vi "S4GUI.vi"(7 "Tab ObsEng":enum32{"Obs", "CCD modes", "Eng"}(tab)) -> ()   [LabVIEW 2018] (continued)
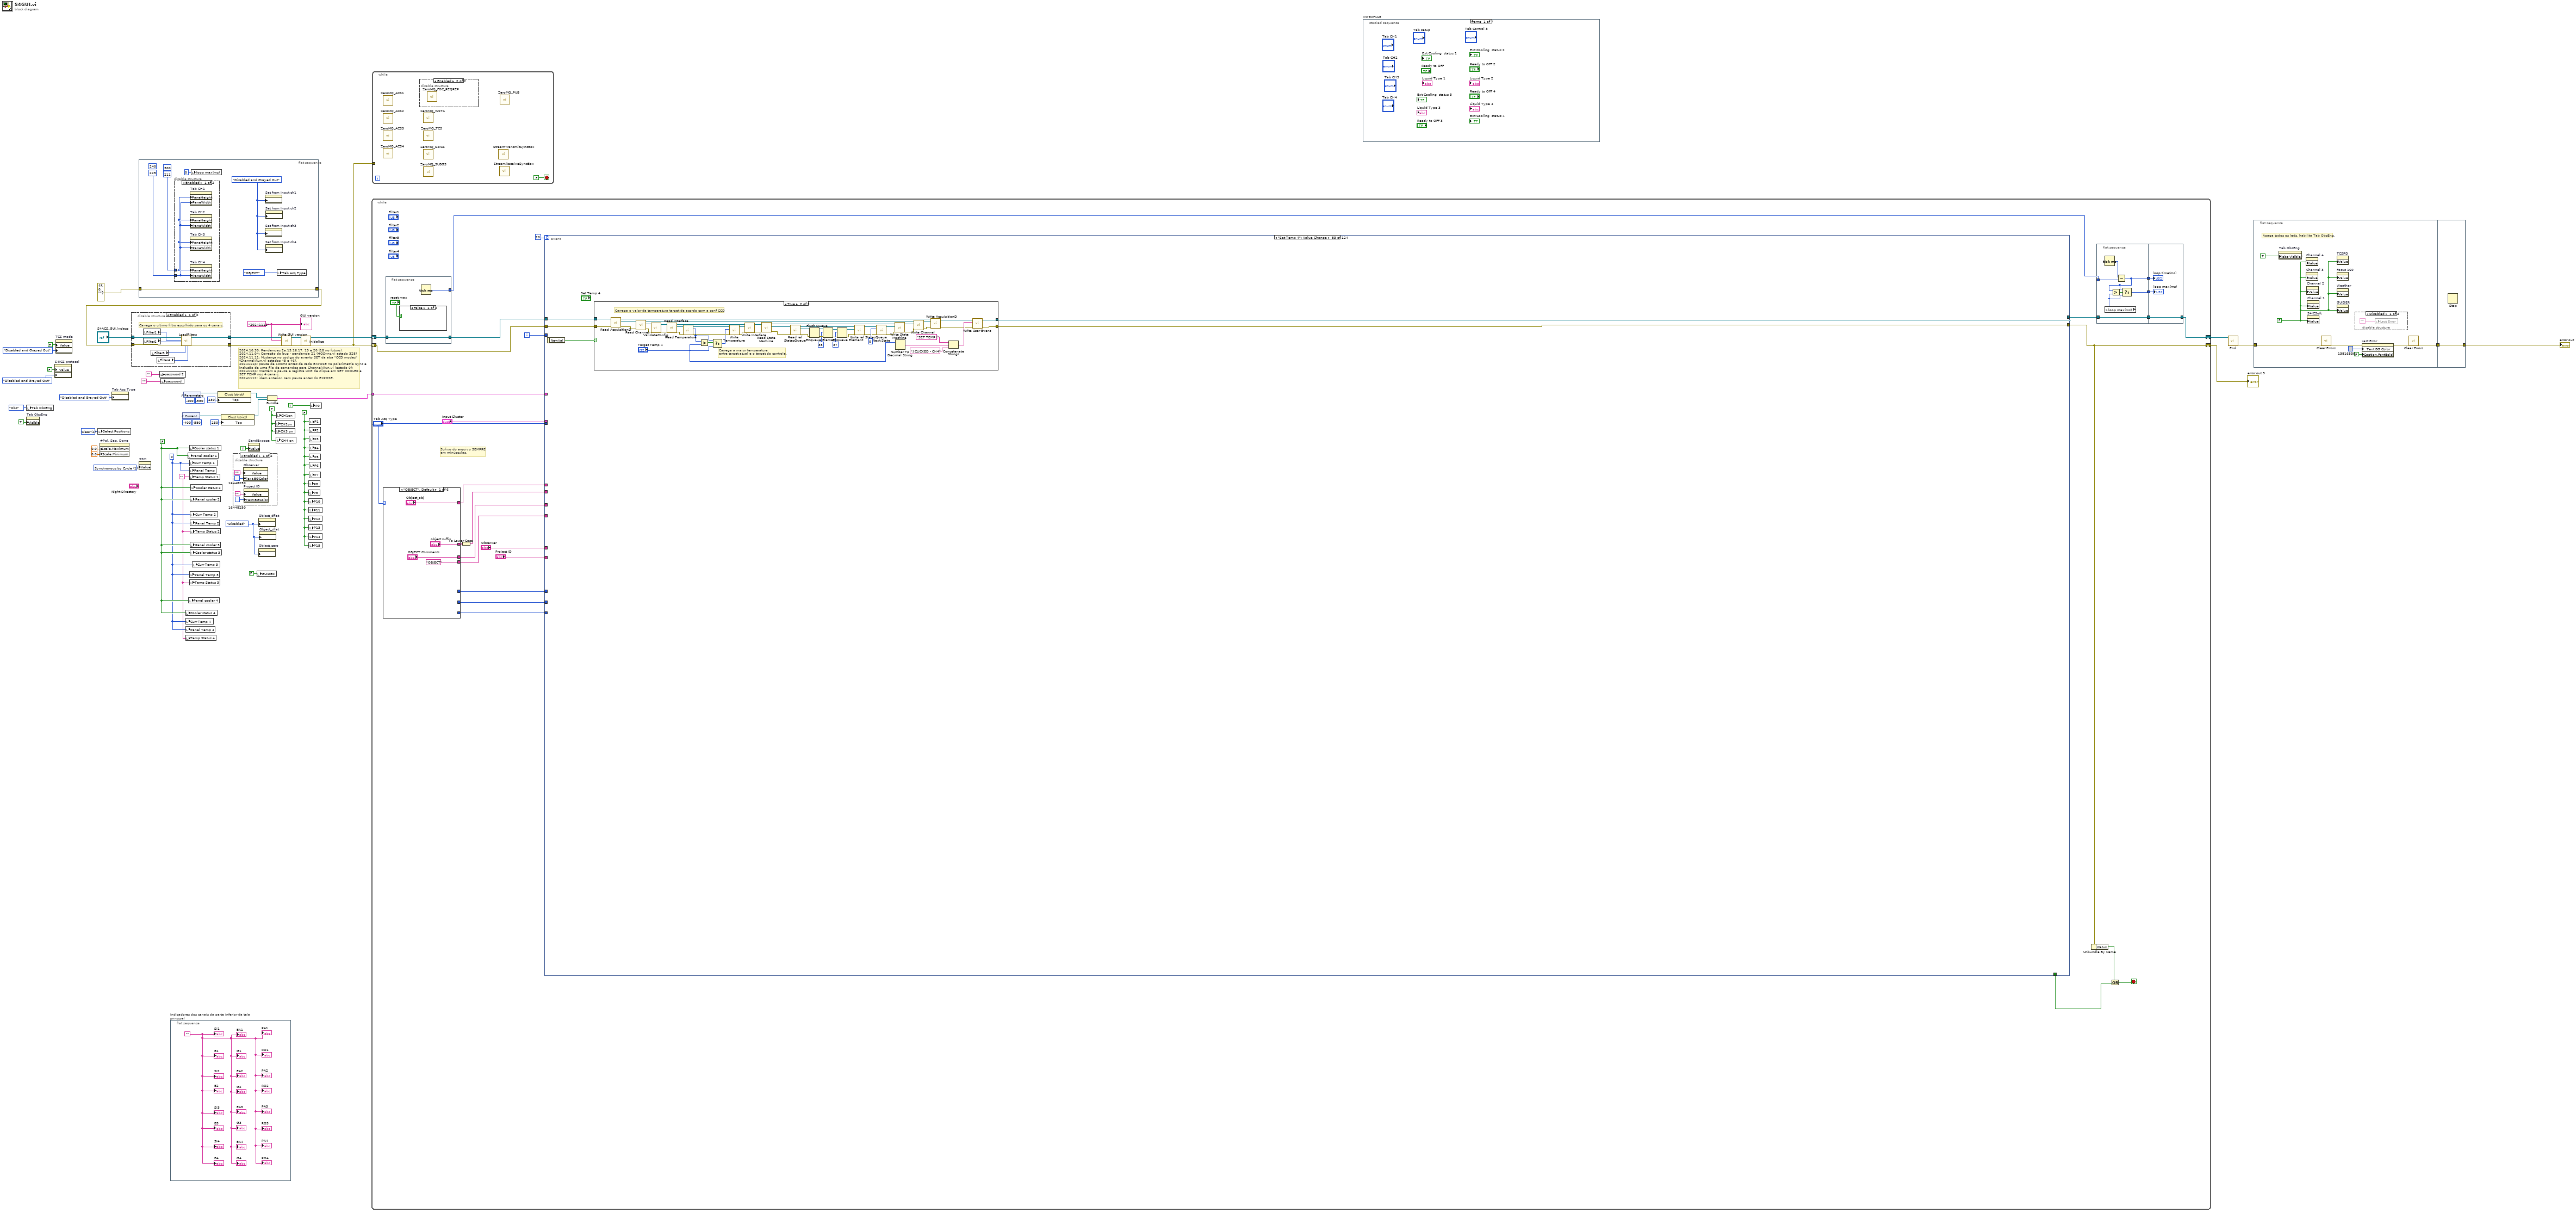
[diagram p0: block diagram]
diagram:
  w11 = "20241112" ("GUI version")
  w21 = TRUE ("CH1on")
  w26 = T12."Disabled" ("Disabled")
  (unwired) -580 ("Position:Top")
  (unwired) -400 ("Position:Top")
  w31 = "" ("Temp Status 1")
  w32 = i16 0 ("Curr Temp 1")
  w33 = FALSE ("Cooler status 1")
  w34 = u16 1 items=["Asynchronous", "Synchronous by Cycle"] ("SSM")
  (unwired) -400 ("Position:Top")
  (unwired) -580 ("Position:Top")
  w43 = u16 4 items=["All 16 positions", "First 8 positions", "First 4 positions", "1-4 & 9-12", "Clear", "Customized"] ("Select Positions")
  w25 = FALSE
  # "2024.10.30: Pendencias 2a,15,16,17, 19 e 20 (18 no futuro).\n2024.11.04: Correção do bug - pendencia 21 (HOSync.vi estado 328)\n2024.11.11: Mudança no código do evento SET da aba \"CCD modes\" \n(Channel:Run.vi estados 45 e 46).\n2024111p: pause de 100ms antes de cada EXPOSE na polarimetria Sync e \ninclusão de uma fila de comandos para Channel:Run.vi (estado 0);\n2024112p: mantém a pausa e registra LOG de clique em SET COOLER e \nSET TEMP nos 4 canais.\n20241112: idem anterior, sem pausa antes do EXPOSE."
  n1 = local write "Tab ObsEng"(enum32{"Obs", "CCD modes", "Eng"}."Obs" ("Tab ObsEng")) -> ()
  n2 = property on="Tab ObsEng" class="TabCtl (strict)"("Visible"=TRUE) -> ()  [unwired: 2 in, 2 out]
  n3 = property on="S4ICS protocol" class="Bool (strict)"("Value"=FALSE ("S4ICS protocol"), "DisabledEnum"=T12."Disabled and Grayed Out" ("Disabled")) -> ()  [unwired: 2 in, 2 out]
  n4 = property on="TCS mode" class="Bool (strict)"("Value"=TRUE ("TCS mode"), "DisabledEnum"=T12."Disabled and Grayed Out" ("Disabled")) -> ()  [unwired: 2 in, 2 out]
  n5 = local write "Select Positions"(w43) -> ()
  n6 = property on="#Pol. Seq. Done" class="Slide (strict)"("Scale.Maximum"=0.0 ("Scale.Range:Maximum"), "Scale.Minimum"=0.0 ("Scale.Range:Minimum")) -> ()  [unwired: 2 in, 2 out]
  n7 = property on="Tab Acq Type" class="TabCtl (strict)"("DisabledEnum"=T12."Disabled and Grayed Out" ("Disabled")) -> ()  [unwired: 2 in, 2 out]
  n8 = disable-structure shown="Enabled" {
    disable-tunnel: "S4ACS_GUI.lvclass" -> [w52 w54]
    disable-tunnel: w28 -> [w51 w53]
    disable-tunnel: [w46 w54] -> w15
    disable-tunnel: [w45 w53] -> w14
    frame Enabled {
      # "Carrega o ultimo filtro escolhido para os 4 canais."
      n9 = local read "Filter1"() -> (w50:u8)
      n10 = local read "Filter2"() -> (w49:u8)
      n11 = local read "Filter3"() -> (w48:u8)
      n12 = local read "Filter4"() -> (w47:u8)
      n13 = call-dynamic "LoadFilters.vi"("Filter 4"=w47, "Filter 3"=w48, "error in (no error)"=w51, "Filter 2"=w49, "Filter 1"=w50, "S4GUI in"=w52) -> ("error out"=w45:errorcluster, "S4GUI out"=w46:refnum<class "S4GUI.lvclass">)  [unwired: 4 in]
    }
    frame Disabled {
    }
  }
  n14 = flat-sequence {
    tunnel: errorcluster {"status"=FALSE, "code"=0, "source"=""} ("error in (no error)") -> [w57]
    tunnel: [w57] -> w28
    frame #0 {
      w56 = T12."Disabled and Grayed Out" ("Disabled")
      (unwired) u32 240 ("Tab Control Pane Dimension:Width")
      (unwired) u32 300 ("Tab Control Pane Dimension:Height")
      n15 = disable-structure shown="Enabled" {
        disable-tunnel: u32 211 ("Tab Control Pane Dimension:Height") -> [w62 _]
        disable-tunnel: u32 225 ("Tab Control Pane Dimension:Width") -> [w61 _]
        frame Enabled {
          n16 = property on="Tab CH1" class="TabCtl (strict)"("PaneHeight"=w62, "PaneWidth"=w61) -> ()  [unwired: 2 in, 2 out]
          n17 = property on="Tab CH2" class="TabCtl (strict)"("PaneHeight"=w62, "PaneWidth"=w61) -> ()  [unwired: 2 in, 2 out]
          n18 = property on="Tab CH3" class="TabCtl (strict)"("PaneHeight"=w62, "PaneWidth"=w61) -> ()  [unwired: 2 in, 2 out]
          n19 = property on="Tab CH4" class="TabCtl (strict)"("PaneHeight"=w62, "PaneWidth"=w61) -> ()  [unwired: 2 in, 2 out]
        }
        frame Disabled {
        }
      }
      n20 = local write "loop max(ms)"(u32 0 ("loop max(ms)")) -> ()
      n21 = property on="Set from Input ch1" class="Bool"("DisabledEnum"=w56) -> ()  [unwired: 2 in, 2 out]
      n22 = property on="Set from Input ch3" class="Bool"("DisabledEnum"=w56) -> ()  [unwired: 2 in, 2 out]
      n23 = property on="Set from Input ch2" class="Bool"("DisabledEnum"=w56) -> ()  [unwired: 2 in, 2 out]
      n24 = property on="Set from Input ch4" class="Bool"("DisabledEnum"=w56) -> ()  [unwired: 2 in, 2 out]
      n25 = local write "Tab Acq Type"(T1."OBJECT" ("Tab Acq Type")) -> ()
    }
  }
  n26 = property on="SSM" class="Ring (strict)"("Value"=w34) -> ()  [unwired: 2 in, 2 out]
  n27 = local write "password 2"("" ("password")) -> ()
  n28 = local write "password"("" ("password")) -> ()
  n29 = flat-sequence "Indicadores dos canais da parte inferior da tela principal" {
    frame #0 {
      w63 = ""
      "B1" <- w63
      "PA1" <- w63
      "RO1" <- w63
      "G1" <- w63
      "SI2" <- w63
      "PA2" <- w63
      "G2" <- w63
      "B2" <- w63
      "RO2" <- w63
      "EA2" <- w63
      "SI3" <- w63
      "EA3" <- w63
      "PA3" <- w63
      "B3" <- w63
      "G3" <- w63
      "RO3" <- w63
      "SI4" <- w63
      "EA4" <- w63
      "PA4" <- w63
      "B4" <- w63
      "G4" <- w63
      "RO4" <- w63
      "SI1" <- w63
      "EA1" <- w63
    }
  }
  n30 = control-ref of="Current Configuration"() -> (w41:refnum<vi>)
  n31 = control-ref of="Parameters"() -> (w38:refnum<vi>)
  n32 = local write "Cooler status 4"(w33) -> ()
  n33 = local write "Curr Temp 4"(w32) -> ()
  n34 = local write "Panel Temp 4"(w32) -> ()
  n35 = local write "Temp Status 4"(w31) -> ()
  n36 = local write "Panel cooler 1"(w33) -> ()
  n37 = local write "Panel cooler 4"(w33) -> ()
  n38 = local write "Cooler status 1"(w33) -> ()
  n39 = local write "Curr Temp 1"(w32) -> ()
  n40 = local write "Panel Temp"(w32) -> ()
  n41 = local write "Temp Status 1"(w31) -> ()
  n42 = local write "Panel Temp 3"(w32) -> ()
  n43 = local write "Temp Status 3"(w31) -> ()
  n44 = local write "Panel cooler 2"(w33) -> ()
  n45 = local write "Curr Temp 2"(w32) -> ()
  n46 = local write "Panel Temp 2"(w32) -> ()
  n47 = local write "Temp Status 2"(w31) -> ()
  n48 = local write "Panel cooler 3"(w33) -> ()
  n49 = local write "Cooler status 3"(w33) -> ()
  n50 = local write "Cooler status 2"(w33) -> ()
  n51 = local write "Curr Temp 3"(w32) -> ()
  n52 = property on="Property Node" class="Clust (strict)"(reference=w38, "Top"=230 ("Position:Top")) -> (reference out=w42:refnum<vi>)  [unwired: 1 in, 1 out]
  n53 = property on="Property Node" class="Clust (strict)"(reference=w41, "Top"=230 ("Position:Top")) -> (reference out=w40:refnum<vi>)  [unwired: 1 in, 1 out]
  n54 = disable-structure shown="Enabled" {
    frame Enabled {
      n55 = property on="Observer" class="Str"("Value"="" ("Observer"), "Text.BGColor"=u32 16448250) -> ()  [unwired: 2 in, 2 out]
      n56 = property on="Project ID" class="Str"("Value"="" ("Observer"), "Text.BGColor"=u32 16448250) -> ()  [unwired: 2 in, 2 out]
    }
    frame Disabled {
    }
  }
  n57 = property on="SendExpose" class="Bool (strict)"("Value"=TRUE ("ExtSync")) -> ()  [unwired: 2 in, 2 out]
  n58 = local write "GUIDER"(FALSE ("GUIDER")) -> ()
  n59 = property on="Object_dflat" class="Str"("DisabledEnum"=w26) -> ()  [unwired: 2 in, 2 out]
  n60 = property on="Object_zero" class="Str"("DisabledEnum"=w26) -> ()  [unwired: 2 in, 2 out]
  n61 = property on="Object_sflat" class="Str"("DisabledEnum"=w26) -> ()  [unwired: 2 in, 2 out]
  n62 = Bundle("Parameters"=w42, "Current Configuration"=w40) -> (w39:T13)  [unwired: 1 in]
  n63 = local write "CH2on"(w21) -> ()
  n64 = local write "CH3 on"(w21) -> ()
  n65 = local write "CH4 on"(w21) -> ()
  n66 = local write "CH1on"(w21) -> ()
  n67 = call-dynamic "Write GUI version.vi"("error in (no error)"=w14, "GUI version"=w11, "S4GUI in"=w15) -> ("error out"=w12:errorcluster, "S4GUI out"=w13:refnum<class "S4GUI.lvclass">)  [unwired: 7 in]
  n68 = call-dynamic "Initialize.vi"("error in (no error)"=w12, "S4ACS_GUI in"=w13) -> ("error out"=w5:errorcluster, "S4ACS_GUI out"=w6:refnum<class "S4GUI.lvclass">)  [unwired: 8 in]
  n69 = local write "P8"(w25) -> ()
  n70 = local write "P9"(w25) -> ()
  n71 = local write "P10"(w25) -> ()
  n72 = local write "P11"(w25) -> ()
  n73 = local write "P12"(w25) -> ()
  n74 = local write "P13"(w25) -> ()
  n75 = local write "P14"(w25) -> ()
  n76 = local write "P15"(w25) -> ()
  n77 = local write "P1"(w25) -> ()
  n78 = local write "P2"(w25) -> ()
  n79 = local write "P3"(w25) -> ()
  n80 = local write "P4"(w25) -> ()
  n81 = local write "P5"(w25) -> ()
  n82 = local write "P6"(w25) -> ()
  n83 = local write "P7"(w25) -> ()
  n84 = local write "P0"(TRUE ("P0")) -> ()
  n85 = while {
    shift-right: [w84] -> w44
    shift-left: w6 -> [w87]
    shift-right: [w71] -> w20
    shift-left: w5 -> [w95]
    tunnel: w39 -> [w92]
    i -> [w77]
    stop <- w68 stop-if-true
    # "Sufixo do arquivo SEMPRE\nem minúsculas."
    n86 = case shown="\"OBJECT\", Default" "Tab Acq Type" {
      tunnel: ["object suffix" "dflat suffix" "sflat suffix" "dark suffix" "zero suffix" "focus suffix"] -> w79
      tunnel: ["OBJECT Comments" "DFLAT Comments" "SFLAT Comments" "DARK Comments" "ZERO Comments" "FOCUS Comments"] -> w93
      tunnel: ["OBJECT" "FLAT" "FLAT" "DARK" "ZERO" "FOCUS"] -> w90
      tunnel: ["Object_obj" "DOMEFLAT" "SKYFLAT" "Object_dark" "ZERO" "Object_focus"] -> w89
      tunnel: [_ _ _ _ _ "Start focus"] -> w76
      tunnel: [_ _ _ _ _ "Step focus"] -> w74
      tunnel: [_ _ _ _ _ "#steps"] -> w75
      frame "OBJECT", Default {
      }
      frame "DFLAT" {
      }
      frame "SFLAT" {
      }
      frame "DARK" {
      }
      frame "ZERO" {
      }
      frame "FOCUS" {
      }
    }
    n87 = flat-sequence {
      tunnel: w87 -> [w108]
      tunnel: [w108] -> w86
      tunnel: [w107] -> w83
      frame #0 {
        n88 = case shown="False" "reset max" {
          frame False {
          }
          frame True {
            n89 = local write "loop max(ms)"(u32 0 ("loop max(ms)")) -> ()
          }
        }
        n90 = Tick Count (ms)() -> (millisecond timer value=w107:u32)
      }
    }
    n91 = To Lower Case(string=w79) -> (all lower case string=w78:string)
    n92 = event shown="[82] \"Set Temp 4\": Value Change" {
      selector: _ -> [_ _ _ _ _ _ _ _ _ _ _ _ _ _ _ _ _ _ _ _ _ _ _ _ _ _ _ _ _ _ _ _ _ _ _ _ _ _ _ _ _ _ _ _ _ _ _ _ _ _ _ _ _ _ _ _ _ _ _ _ _ _ _ _ _ _ _ _ _ _ _ _ _ _ _ _ _ _ _ _ _ _ _ _ _ _ _ _ _ _ _ _ _ _ _ _ _ _ _ _ _ _ _ _ _ _ _ _ _ _ _ _ _ _ _ _ _ _ _ _ _ _ _ _]
      dyn-events: _ -> [_ _ _ _ _ _ _ _ _ _ _ _ _ _ _ _ _ _ _ _ _ _ _ _ _ _ _ _ _ _ _ _ _ _ _ _ _ _ _ _ _ _ _ _ _ _ _ _ _ _ _ _ _ _ _ _ _ _ _ _ _ _ _ _ _ _ _ _ _ _ _ _ _ _ _ _ _ _ _ _ _ _ _ _ _ _ _ _ _ _ _ _ _ _ _ _ _ _ _ _ _ _ _ _ _ _ _ _ _ _ _ _ _ _ _ _ _ _ _ _ _ _ _ _]
      timeout: 20 -> [_ _ _ _ _ _ _ _ _ _ _ _ _ _ _ _ _ _ _ _ _ _ _ _ _ _ _ _ _ _ _ _ _ _ _ _ _ _ _ _ _ _ _ _ _ _ _ _ _ _ _ _ _ _ _ _ _ _ _ _ _ _ _ _ _ _ _ _ _ _ _ _ _ _ _ _ _ _ _ _ _ _ _ _ _ _ _ _ _ _ _ _ _ _ _ _ _ _ _ _ _ _ _ _ _ _ _ _ _ _ _ _ _ _ _ _ _ _ _ _ _ _ _ _]
      tunnel: w86 -> [w179 w2139 w2298 w2328 w2334 w2356 w2378 w2549 w2557 w2636 w2657 w2729 w2800 w2901 w2916 w3042 w3221 w3253 w3285 w3317 w3352 w3387 w3422 w3457 w3460 w3494 w3636 w3697 w4204 w4283 w4355 w4426 w4499 w4550 w4591 w5020 w5026 w5141 w6423 w6694 w6899 w7100 w7313 w7532 w7547 w7755 w7917 w8084 w8251 w8410 w8430 w8450 w8470 w8491 w8556 w8621 w8686 w8751 w8788 w8816 w8844 w8873 w8946 w9076 w9110 w9169 w9228 w9287 w9346 w9366 w9393 w9409 w9430 w9460 w9490 w9520 w9555 w9594 w9634 w9673 w9734 w9795 w9856 w9922 w9942 w9957 w9972 w9987 w10002 w10017 w10032 w10047 w10078 w10107 w10131 w10173 w10207 w10234 w10257 w10285 w10305 w10320 w10340 w10423 w10751 w10782 w10842 w10862 w10877 w10897 w10917 w10937 w10952 w10972 w10992 w11012 w11027 w11047 w11067 w11087 w11102 w11122 w11142 w11162]
      tunnel: w95 -> [w178 w2140 w2296 w2327 w2333 w2355 w2377 w2548 w2556 w2635 w2656 w2728 w2801 w2900 w2907 w3033 w3220 w3252 w3284 w3316 w3351 w3386 w3421 w3456 w3468 w3495 w3635 w3696 w4203 w4282 w4354 w4422 w4498 w4548 w4590 w5019 w5025 w5140 w6422 w6693 w6898 w7099 w7306 w7530 w7546 w7753 w7916 w8082 w8250 w8411 w8431 w8451 w8471 w8490 w8555 w8620 w8685 w8749 w8786 w8814 w8842 w8872 w8945 w9075 w9109 w9168 w9227 w9286 w9345 w9365 w9392 w9408 w9429 w9459 w9489 w9518 w9554 w9593 w9633 w9672 w9733 w9794 w9855 w9921 w9941 w9956 w9971 w9986 w10001 w10016 w10031 w10046 w10077 w10106 w10130 w10172 w10206 w10233 w10256 w10284 w10304 w10319 w10339 w10424 w10750 w10781 w10841 w10861 w10876 w10896 w10916 w10936 w10951 w10971 w10991 w11011 w11026 w11046 w11066 w11086 w11101 w11121 w11141 w11161]
      tunnel: [w139 w2102 w2290 w2315 w2335 w2357 w2379 w2536 w2574 w2635 w2674 w2746 w2818 w2887 w2914 w3040 w3131 w3239 w3271 w3303 w3342 w3377 w3412 w3447 w3468 w3480 w3600 w3684 w4123 w4280 w4352 w4417 w4496 w4551 w4585 w5018 w5022 w5106 w6484 w6687 w6892 w7093 w7307 w7531 w7539 w7749 w7926 w8093 w8260 w8409 w8429 w8449 w8469 w8489 w8554 w8619 w8684 w8750 w8787 w8815 w8843 w8877 w8950 w9077 w9108 w9167 w9226 w9285 w9344 w9364 w9391 w9407 w9428 w9458 w9488 w9547 w9585 w9624 w9663 w9671 w9732 w9793 w9854 w9920 w9940 w9955 w9970 w9985 w10000 w10015 w10030 w10045 w10062 w10104 w10129 w10171 w10205 w10232 w10255 w10267 w10287 w10307 w10323 w10347 w10758 w10783 w10824 w10844 w10864 w10882 w10899 w10919 w10939 w10955 w10974 w10994 w11014 w11030 w11049 w11069 w11089 w11105 w11124 w11144] -> w71
      tunnel: [w138 _ _ _ _ _ _ _ _ _ _ _ _ _ _ _ _ _ _ _ _ _ _ _ _ _ _ _ _ _ _ _ _ _ _ _ _ _ _ _ _ _ _ _ _ _ _ _ _ _ _ _ _ _ _ _ _ _ _ _ _ _ _ _ _ _ _ _ _ _ _ _ _ _ _ _ _ _ _ _ _ _ _ _ _ _ _ _ _ _ _ _ _ _ _ _ _ _ _ _ _ _ _ _ _ _ _ _ _ _ _ _ _ _ _ _ _ _ _ _ _ _ _ _] -> w69
      tunnel: w78 -> [_ _ _ _ _ _ _ _ _ _ _ _ _ _ _ _ _ _ _ _ _ _ _ _ _ _ _ _ _ _ _ _ _ _ w4584 _ _ _ _ w6692 w6896 _ w7311 _ w7544 w7762 w7925 w8092 w8259 _ _ _ _ _ _ _ _ _ _ _ _ _ _ _ _ _ _ _ _ _ _ _ _ _ _ _ _ _ _ _ _ _ _ _ _ _ _ _ _ _ _ _ _ _ _ _ _ _ _ _ _ _ _ _ _ _ _ _ _ _ _ _ _ _ _ _ _ _ _ _ _ _ _ _]
      tunnel: w93 -> [_ _ _ _ _ _ _ _ _ _ _ _ _ _ _ _ _ _ _ _ _ _ _ _ _ _ _ _ _ _ _ _ _ _ w4583 _ _ _ _ w6691 _ w7097 w7310 _ w7543 w7761 w7924 w8091 w8258 _ _ _ _ _ _ _ _ _ _ _ _ _ _ _ _ _ _ _ _ _ _ _ _ _ _ _ _ _ _ _ _ _ _ _ _ _ _ _ _ _ _ _ _ _ _ _ _ _ _ _ _ _ _ _ _ _ _ _ _ _ _ _ _ _ _ _ _ _ _ _ _ _ _ _]
      tunnel: w92 -> [_ _ _ _ _ _ _ _ _ _ _ _ _ _ _ _ _ _ _ _ _ _ _ _ w3461 _ _ _ _ _ _ _ _ _ _ _ _ _ _ _ _ _ _ _ _ _ _ _ _ _ _ _ _ _ _ _ _ _ _ _ _ _ _ _ _ _ _ _ _ _ _ _ _ _ _ _ _ _ _ _ _ _ _ _ _ _ _ _ _ _ _ _ _ _ _ _ _ _ _ _ _ _ _ _ _ _ _ _ _ _ _ _ _ _ _ _ _ _ _ _ _ _ _ _]
      tunnel: [w140 w2104 w2289 w2316 w2336 w2358 w2380 w2537 w2575 w2636 w2675 w2747 w2819 w2878 w2915 w3041 w3133 w3230 w3262 w3294 w3319 w3354 w3389 w3424 w3460 w3479 w3601 w3685 w4124 w4281 w4353 w4418 w4497 w4552 w4565 w5017 w5021 w5107 w6483 w6688 w6893 w7094 w7308 w7532 w7540 w7750 w7923 w8090 w8257 w8408 w8428 w8448 w8468 w8488 w8553 w8618 w8683 w8748 w8785 w8813 w8841 w8875 w8948 w9078 w9107 w9166 w9225 w9284 w9343 w9363 w9383 w9406 w9427 w9457 w9487 w9546 w9586 w9625 w9664 w9670 w9731 w9792 w9853 w9913 w9936 w9951 w9966 w9981 w9996 w10011 w10026 w10041 w10061 w10079 w10116 w10140 w10188 w10218 w10243 w10266 w10286 w10306 w10321 w10348 w10759 w10784 w10823 w10843 w10863 w10880 w10898 w10918 w10938 w10953 w10973 w10993 w11013 w11028 w11048 w11068 w11088 w11103 w11123 w11143] -> w85
      tunnel: "Input Cluster" -> [_ _ _ _ _ _ _ _ _ _ _ _ _ _ _ _ _ _ _ _ _ _ _ _ w3459 _ _ _ _ _ _ _ _ _ _ _ _ _ _ _ _ _ _ _ _ _ _ _ _ _ _ _ _ _ _ _ _ _ _ _ _ _ _ _ _ _ _ _ _ _ _ _ _ _ _ _ _ _ _ _ _ _ _ _ _ _ _ _ _ _ _ _ _ _ _ _ _ _ _ _ _ _ _ _ _ _ _ _ _ _ _ _ _ _ _ _ _ _ _ _ _ _ _ _]
      tunnel: w90 -> [_ _ _ _ _ _ _ _ _ _ _ _ _ _ _ _ _ _ _ _ _ _ _ _ _ _ _ _ _ _ _ _ _ _ w4582 _ _ _ _ w6689 w6894 w7095 w7309 _ w7541 w7760 w7922 w8088 w8256 _ _ _ _ _ _ _ _ _ _ _ _ _ _ _ _ _ _ _ _ _ _ _ _ _ _ _ _ _ _ _ _ _ _ _ _ _ _ _ _ _ _ _ _ _ _ _ _ _ _ _ _ _ _ _ _ _ _ _ _ _ _ _ _ _ _ _ _ _ _ _ _ _ _ _]
      tunnel: w89 -> [_ _ _ _ _ _ _ _ _ _ _ _ _ _ _ _ _ _ _ _ _ _ _ _ _ _ _ _ _ _ _ _ _ _ w4581 _ _ _ _ _ w6897 w7098 w7312 _ w7545 w7759 w7921 w8089 w8255 _ _ _ _ _ _ _ _ _ _ _ _ _ _ _ _ _ _ _ _ _ _ _ _ _ _ _ _ _ _ _ _ _ _ _ _ _ _ _ _ _ _ _ _ _ _ _ _ _ _ _ _ _ _ _ _ _ _ _ _ _ _ _ _ _ _ _ _ _ _ _ _ _ _ _]
      tunnel: "Observer" -> [_ _ _ _ _ _ _ _ _ _ _ _ _ _ _ _ _ _ _ _ _ _ _ _ _ _ _ _ _ _ _ _ _ _ w4580 _ _ w5112 w6432 w6690 w6895 w7096 _ _ w7542 w7758 w7920 w8087 w8254 _ _ _ _ _ _ _ _ _ _ _ _ _ _ _ _ _ _ _ _ _ _ _ _ _ _ _ _ _ _ _ _ _ _ _ _ _ _ _ _ _ _ _ _ _ _ _ _ _ _ _ _ _ _ _ _ _ _ _ _ _ _ _ _ _ _ _ _ _ _ _ _ _ _ _]
      tunnel: w77 -> [w159 _ _ _ _ _ _ _ _ _ _ _ _ _ _ _ _ _ _ _ _ _ _ _ _ _ _ _ _ _ _ _ _ _ _ _ _ _ _ _ _ _ _ _ _ _ _ _ _ _ _ _ _ _ _ _ _ _ _ _ _ _ _ _ _ _ _ _ _ _ _ _ _ _ _ _ _ _ _ _ _ _ _ _ _ _ _ _ _ _ _ _ _ _ _ _ _ _ _ _ _ _ _ _ _ _ _ _ _ _ _ _ _ _ _ _ _ _ _ _ _ _ _ _]
      tunnel: "Tab Acq Type" -> [_ _ _ _ _ _ _ _ _ _ _ _ _ _ _ _ _ _ _ _ _ _ _ _ _ _ _ _ _ _ _ _ _ _ w4572 _ _ _ _ _ _ w7084 _ _ _ w7747 w7911 w8078 w8244 _ _ _ _ _ _ _ _ _ _ _ _ _ _ _ _ _ _ _ _ _ _ _ _ _ _ _ _ _ _ _ _ _ _ _ _ _ _ _ _ _ _ _ _ _ _ _ _ _ _ _ _ _ _ _ _ _ _ _ _ _ _ _ _ _ _ _ _ _ _ _ _ _ _ _]
      tunnel: w76 -> [_ _ _ _ _ _ _ _ _ _ _ _ _ _ _ _ _ _ _ _ _ _ _ _ _ _ _ _ _ _ _ _ _ _ w4571 _ _ _ _ _ _ _ _ _ _ w7746 w7910 w8077 w8243 _ _ _ _ _ _ _ _ _ _ _ _ _ _ _ _ _ _ _ _ _ _ _ _ _ _ _ _ _ _ _ _ _ _ _ _ _ _ _ _ _ _ _ _ _ _ _ _ _ _ _ _ _ _ _ _ _ _ _ _ _ _ _ _ _ _ _ _ _ _ _ _ _ _ _]
      tunnel: w75 -> [_ _ _ _ _ _ _ _ _ _ _ _ _ _ _ _ _ _ _ _ _ _ _ _ _ _ _ _ _ _ _ _ _ _ w4569 _ _ _ _ _ _ _ _ _ _ w7744 w7908 w8075 w8241 _ _ _ _ _ _ _ _ _ _ _ _ _ _ _ _ _ _ _ _ _ _ _ _ _ _ _ _ _ _ _ _ _ _ _ _ _ _ _ _ _ _ _ _ _ _ _ _ _ _ _ _ _ _ _ _ _ _ _ _ _ _ _ _ _ _ _ _ _ _ _ _ _ _ _]
      tunnel: w74 -> [_ _ _ _ _ _ _ _ _ _ _ _ _ _ _ _ _ _ _ _ _ _ _ _ _ _ _ _ _ _ _ _ _ _ w4570 _ _ _ _ _ _ _ _ _ _ w7745 w7909 w8076 w8242 _ _ _ _ _ _ _ _ _ _ _ _ _ _ _ _ _ _ _ _ _ _ _ _ _ _ _ _ _ _ _ _ _ _ _ _ _ _ _ _ _ _ _ _ _ _ _ _ _ _ _ _ _ _ _ _ _ _ _ _ _ _ _ _ _ _ _ _ _ _ _ _ _ _ _]
      tunnel: "Project ID" -> [_ _ _ _ _ _ _ _ _ _ _ _ _ _ _ _ _ _ _ _ _ _ _ _ _ _ _ _ _ _ _ _ _ _ _ _ _ w5111 w6431 _ _ _ _ _ _ _ _ _ _ _ _ _ _ _ _ _ _ _ _ _ _ _ _ _ _ _ _ _ _ _ _ _ _ _ _ _ _ _ _ _ _ _ _ _ _ _ _ _ _ _ _ _ _ _ _ _ _ _ _ _ _ _ _ _ _ _ _ _ _ _ _ _ _ _ _ _ _ _ _ _ _ _ _ _]
      event Timeout {
        # "2024.07.02: Mostra as publicações das aplicações."
        # "Trata as tarefas para atender \naos clientes: Publisher"
        # "Conteudo dos indicadores"
        # "Status dos indicadores: Habilitado ou Desab."
        # "Obtém os valores de status dos\ndispositivos de cada servidor para\napresentar nos indicadores da GUI."
        # "Trata as tarefas individuais de \ncada servidor (ACS1,...,ACS4, \nICS, TCS, Focus,Weather)"
        # "Determina a sequência de\ntarefas dos servidores\npara uma observação, de \nacordo com o modo de \noperação (disparado com \nos botões START)"
        # "execução dos botões\n no modo sincrono."
        # "execução dos botões\n no modo assincrono."
        n93 = event-data() -> ()  [unwired: 1 in, 2 out]
        n94 = disable-structure shown="Enabled" {
          disable-tunnel: w179 -> [w185 w190]
          disable-tunnel: w178 -> [w184 w188]
          disable-tunnel: [w182 w187] -> w153
          disable-tunnel: [w181 w186] -> w152
          disable-tunnel: w159 -> [_ w189]
          frame Disabled {
            n95 = call "Elapsed Time"() -> ("Time has Elapsed"=w180:bool)  [unwired: 12 in, 7 out]
            n96 = call "Elapsed Time3"() -> ("Time has Elapsed"=w183:bool)  [unwired: 12 in, 7 out]
            n97 = call "Write Status_timeout.vi"("error in (no error)"=w184, "TCS_timeout"=w183, "Status_timeout"=w180, "S4ACS_GUI in"=w185) -> ("error out"=w182:errorcluster, "S4ACS_GUI out"=w181:refnum<class "S4GUI.lvclass">)  [unwired: 6 in]
          }
          frame Enabled {
            n98 = call-dynamic "Write loop counter.vi"("error in (no error)"=w188, "loop counter"=w189, "S4GUI in"=w190) -> ("error out"=w187:errorcluster, "S4GUI out"=w186:refnum<class "S4GUI.lvclass">)  [unwired: 7 in]
          }
        }
        n99 = call-dynamic "GetPubs.vi"("error in (no error)"=w153, "S4GUI in"=w152) -> ("error out"=w154:errorcluster, "Pubs out"=→"All Pubs":T11, "S4GUI out"=w151:refnum<class "S4GUI.lvclass">)  [unwired: 7 in]
        n100 = call-dynamic "HandlePauseAsync.vi"("error in (no error)"=w154, "S4GUI in"=w151) -> ("error out"=w172:errorcluster, "S4GUI out"=w174:refnum<class "S4GUI.lvclass">)  [unwired: 8 in]
        n101 = call-dynamic "HandleStopAsync.vi"("error in (no error)"=w172, "S4GUI in"=w174) -> ("error out"=w171:errorcluster, "S4GUI out"=w173:refnum<class "S4GUI.lvclass">)  [unwired: 8 in]
        n102 = call-dynamic "HandleAbortAsync.vi"("error in (no error)"=w171, "S4GUI in"=w173) -> ("error out"=w165:errorcluster, "S4GUI out"=w166:refnum<class "S4GUI.lvclass">)  [unwired: 8 in]
        n103 = call-dynamic "HandlePauseSync.vi"("error in (no error)"=w165, "S4GUI in"=w166) -> ("error out"=w164:errorcluster, "S4GUI out"=w163:refnum<class "S4GUI.lvclass">)  [unwired: 8 in]
        n104 = call-dynamic "HandleStopSync.vi"("error in (no error)"=w164, "S4GUI in"=w163) -> ("error out"=w168:errorcluster, "S4GUI out"=w170:refnum<class "S4GUI.lvclass">)  [unwired: 8 in]
        n105 = call-dynamic "HandleAbortSync.vi"("error in (no error)"=w168, "S4GUI in"=w170) -> ("error out"=w167:errorcluster, "S4GUI out"=w169:refnum<class "S4GUI.lvclass">)  [unwired: 8 in]
        n106 = call-dynamic "HandleObservation.vi"("error in (no error)"=w167, "S4ACS_GUI in"=w169) -> ("error out"=w176:errorcluster, "S4ACS_GUI out"=w177:refnum<class "S4GUI.lvclass">)  [unwired: 8 in]
        n107 = call-dynamic "HandleServers.vi"("error in (no error)"=w176, "S4GUI in"=w177) -> ("error out"=w157:errorcluster, "S4GUI out"=w158:refnum<class "S4GUI.lvclass">)  [unwired: 8 in]
        n108 = call "Elapsed Time2"() -> ("Time has Elapsed"=w162:bool)  [unwired: 12 in, 7 out]
        n109 = call-dynamic "HandleClients.vi"("error in (no error)"=w157, "S4GUI in"=w158) -> ("error out"=w156:errorcluster, "S4GUI out"=w146:refnum<class "S4GUI.lvclass">)  [unwired: 8 in]
        n110 = call-dynamic "GetStatus.vi"("error in (no error)"=w156, "S4GUI in"=w146) -> ("error out"=w148:errorcluster, "S4GUI out"=w145:refnum<class "S4GUI.lvclass">)  [unwired: 8 in]
        n111 = call-dynamic "Read output cluster.vi"("error in (no error)"=w148, "S4GUI in"=w145) -> ("error out"=w147:errorcluster, "output cluster"=w137:T15, "S4GUI out"=w144:refnum<class "S4GUI.lvclass">)  [unwired: 7 in]
        n112 = call-dynamic "Read Cluster Disable.vi"("error in (no error)"=w147, "S4GUI in"=w144) -> ("error out"=w149:errorcluster, "Cluster Disable"=w150:T16, "S4GUI out"=w143:refnum<class "S4GUI.lvclass">)  [unwired: 7 in]
        n113 = call "Read cfg file.vi"("error in (no error)"=w149, "S4ACS_GUI in"=w143) -> ("error out"=w160:errorcluster, "cfg file"=w175:string, "S4ACS_GUI out"=w161:refnum<class "S4GUI.lvclass">)  [unwired: 7 in]
        n114 = case shown="True" w162 {
          tunnel: w137 -> [_ w244]
          tunnel: w150 -> [_ w243]
          tunnel: w175 -> [_ w242]
          tunnel: w161 -> [w192 w241]
          tunnel: w160 -> [w191 w240]
          tunnel: [w192 w203] -> w142
          tunnel: [w191 w202] -> w141
          frame False {
          }
          frame True {
            w197 = "Parking" ("regular expression")
            w217 = "ERRO" ("regular expression")
            # "Verifica mudança de modo e se deve carregar valores default \npara procedimento de ajuste de foco do telescópio."
            # "1a vez FOTOM (F)"
            # "1a vez POLAR (F)"
            # "MODE:\nF -> photometric\nT -> polarimetric"
            n115 = stacked-sequence {
              tunnel: w241 -> [w293 w300 w311 w321 w330]
              tunnel: w240 -> [w292 w299 w310 w320 w329]
              tunnel: [_ _ _ _ w328] -> w234
              tunnel: [_ _ _ _ w327] -> w233
              tunnel: [_ _ _ _ w326] -> w200
              frame #0 {
                n116 = call-dynamic "Read AcquisitionA.vi"("error in (no error)"=w292, "S4ACS_GUI in"=w293) -> ("error out"=w289:errorcluster, "Acquisition.lvclass"=w291:refnum<class "Acquisition.lvclass">)  [unwired: 7 in, 1 out]
                n117 = call-dynamic "Read Channel.vi"("error in (no error)"=w289, "Acquisition in"=w291) -> ("error out"=w288:errorcluster, "Channel.lvclass"=w290:refnum<class "Channel.lvclass">)  [unwired: 7 in, 1 out]
                n118 = call-dynamic "Read CyclesDone.vi"("error in (no error)"=w288, "Channel in"=w290) -> ("error out"=→"error out 6":errorcluster, "CyclesDone"=w285:u32)  [unwired: 7 in, 1 out]
                "Cycles Done ch1" <- w285
                n119 = Number To Decimal String(number=w285) -> (decimal integer string=w284:string)  [unwired: 1 in]
                n120 = Concatenate Strings("#Cycles Done ", w284) -> (w283:string)
                n121 = property on="Cycles Done ch1" class="Slide (strict)"("Caption.Text"=w283) -> ()  [unwired: 2 in, 2 out]
              }
              frame #1 {
                n122 = call "Read AcquisitionB.vi"("error in (no error)"=w299, "S4ACS_GUI in"=w300) -> ("error out"=w302:errorcluster, "Acquisition.lvclass"=w303:refnum<class "Acquisition.lvclass">)  [unwired: 7 in, 1 out]
                n123 = call-dynamic "Read Channel.vi"("error in (no error)"=w302, "Acquisition in"=w303) -> ("error out"=w301:errorcluster, "Channel.lvclass"=w304:refnum<class "Channel.lvclass">)  [unwired: 7 in, 1 out]
                n124 = call-dynamic "Read CyclesDone.vi"("error in (no error)"=w301, "Channel in"=w304) -> ("error out"=→"error out 4":errorcluster, "CyclesDone"=w295:u32)  [unwired: 7 in, 1 out]
                "Cycles Done ch2" <- w295
                n125 = Number To Decimal String(number=w295) -> (decimal integer string=w296:string)  [unwired: 1 in]
                n126 = Concatenate Strings("#Cycles Done ", w296) -> (w294:string)
                n127 = property on="Cycles Done ch2" class="Slide (strict)"("Caption.Text"=w294) -> ()  [unwired: 2 in, 2 out]
              }
              frame #2 {
                n128 = call-dynamic "Read AcquisitionC.vi"("error in (no error)"=w310, "S4ACS_GUI in"=w311) -> ("error out"=w313:errorcluster, "Acquisition.lvclass"=w314:refnum<class "Acquisition.lvclass">)  [unwired: 7 in, 1 out]
                n129 = call-dynamic "Read Channel.vi"("error in (no error)"=w313, "Acquisition in"=w314) -> ("error out"=w312:errorcluster, "Channel.lvclass"=w315:refnum<class "Channel.lvclass">)  [unwired: 7 in, 1 out]
                n130 = call-dynamic "Read CyclesDone.vi"("error in (no error)"=w312, "Channel in"=w315) -> ("error out"=→"error out 5":errorcluster, "CyclesDone"=w306:u32)  [unwired: 7 in, 1 out]
                "Cycles Done ch3" <- w306
                n131 = Number To Decimal String(number=w306) -> (decimal integer string=w307:string)  [unwired: 1 in]
                n132 = Concatenate Strings("#Cycles Done ", w307) -> (w305:string)
                n133 = property on="Cycles Done ch3" class="Slide (strict)"("Caption.Text"=w305) -> ()  [unwired: 2 in, 2 out]
              }
              frame #3 {
                n134 = call-dynamic "Read AcquisitionD.vi"("error in (no error)"=w320, "S4ACS_GUI in"=w321) -> ("error out"=w323:errorcluster, "Acquisition.lvclass"=w324:refnum<class "Acquisition.lvclass">)  [unwired: 7 in, 1 out]
                n135 = call-dynamic "Read Channel.vi"("error in (no error)"=w323, "Acquisition in"=w324) -> ("error out"=w322:errorcluster, "Channel.lvclass"=w325:refnum<class "Channel.lvclass">)  [unwired: 7 in, 1 out]
                n136 = call-dynamic "Read CyclesDone.vi"("error in (no error)"=w322, "Channel in"=w325) -> ("CyclesDone"=w317:u32)  [unwired: 7 in, 2 out]
                "Cycles Done ch4" <- w317
                n137 = Number To Decimal String(number=w317) -> (decimal integer string=w318:string)  [unwired: 1 in]
                n138 = Concatenate Strings("#Cycles Done ", w318) -> (w316:string)
                n139 = property on="Cycles Done ch4" class="Slide (strict)"("Caption.Text"=w316) -> ()  [unwired: 2 in, 2 out]
              }
              frame #4 {
                n140 = call-dynamic "Read SET request.vi"("error in (no error)"=w329, "S4GUI in"=w330) -> ("error out"=w327:errorcluster, "SET request"=w326:bool, "S4GUI out"=w328:refnum<class "S4GUI.lvclass">)  [unwired: 7 in]
              }
            }
            n141 = stacked-sequence {
              tunnel: w244 -> [w376 w386 w398 w400 w407 w441 w444 w578 w681 w1023 _ _ _ _ _ w1215 w1401 w1564 w1723 w1826]
              tunnel: [_ _ _ _ _ _ _ w576 _ _ _ _ _ _ _ _ _ _ _ _] -> w224
              tunnel: w243 -> [_ w382 _ _ _ _ _ _ _ _ w1050 w1097 w1114 w1131 w1148 _ _ _ _ _]
              tunnel: w242 -> [_ _ _ _ _ _ _ _ _ _ _ _ _ _ _ w1210 _ _ _ _]
              tunnel: w200 -> [_ _ _ _ _ _ _ _ _ _ _ _ _ _ _ _ _ _ _ w1829]
              frame #0 {
                (unwired) u32 240 ("Tab Control Pane Dimension:Width")
                (unwired) u32 300 ("Tab Control Pane Dimension:Height")
                n142 = Unbundle By Name(w376) -> ("GS STATUS cluster.AG"=→"GUIDER":bool, "TCS id"=w342:u32, "TCSPD_connection"=→"TCSPD":bool, "TCS extended"=w373:string, "focus pos"=w338:i32, "weather status"=w336:T17)
                n143 = Unbundle By Name(w336) -> ("outTemp"=→"Outside Temp":string, "pressure"=→"Pressure":string, "outHumidity"=→"Humidity":string, "windSpeed"=→"Wind Speed[Km/h]":string)
                n144 = Number To Decimal String(number=w338) -> (decimal integer string=→"Telescope Focus":string)  [unwired: 1 in]
                n145 = Equal?(x=u32 6 ("Tab Control Pane Dimension:Width"), y=w342) -> (x = y?=w341:bool)
                n146 = Match Pattern(string=w373, regular expression="RA=") -> (after substring=w369:string)  [unwired: 1 in, 3 out]
                n147 = local write "TCS mode"(w341) -> ()
                n148 = Match Pattern(string=w369, regular expression="DEC=") -> (before substring=→"RA":string, after substring=w368:string)  [unwired: 1 in, 2 out]
                n149 = Match Pattern(string=w368, regular expression="EQUINOX=") -> (before substring=→"DEC":string, after substring=w367:string)  [unwired: 1 in, 2 out]
                n150 = Match Pattern(string=w367, regular expression="AIRMASS=") -> (after substring=w363:string)  [unwired: 1 in, 3 out]
                n151 = Match Pattern(string=w363, regular expression="TCSHA=") -> (before substring=→"Air Mass":string, after substring=w362:string)  [unwired: 1 in, 2 out]
                n152 = Match Pattern(string=w362, regular expression="TCSDATE=") -> (before substring=→"Hour Angle":string, after substring=w360:string)  [unwired: 1 in, 2 out]
                n153 = Match Pattern(string=w360, regular expression="TELFOCUS=") -> (before substring=→"Date":string, after substring=w356:string)  [unwired: 1 in, 2 out]
                n154 = Match Pattern(string=w356, regular expression="EXTTEMP=") -> (after substring=w355:string)  [unwired: 1 in, 3 out]
                n155 = Match Pattern(string=w355, regular expression="PRESSURE=") -> (after substring=w354:string)  [unwired: 1 in, 3 out]
                n156 = Match Pattern(string=w354, regular expression="HUMIDITY=") -> (after substring=w346:string)  [unwired: 1 in, 3 out]
                n157 = Match Pattern(string=w346, regular expression="JD=") -> (after substring=w347:string)  [unwired: 1 in, 3 out]
                n158 = disable-structure shown="Enabled" {
                  disable-tunnel: u32 211 ("Tab Control Pane Dimension:Height") -> [w378 _]
                  disable-tunnel: u32 225 ("Tab Control Pane Dimension:Width") -> [w377 _]
                  frame Disabled {
                    n159 = property on="Tab CH1" class="TabCtl (strict)"("PaneHeight"=w378, "PaneWidth"=w377) -> ()  [unwired: 2 in, 2 out]
                    n160 = property on="Tab CH2" class="TabCtl (strict)"("PaneHeight"=w378, "PaneWidth"=w377) -> ()  [unwired: 2 in, 2 out]
                    n161 = property on="Tab CH3" class="TabCtl (strict)"("PaneHeight"=w378, "PaneWidth"=w377) -> ()  [unwired: 2 in, 2 out]
                    n162 = property on="Tab CH4" class="TabCtl (strict)"("PaneHeight"=w378, "PaneWidth"=w377) -> ()  [unwired: 2 in, 2 out]
                  }
                  frame Enabled {
                  }
                }
                n163 = Match Pattern(string=w347, regular expression="SD=") -> (before substring=→"Julian Date":string, after substring=→"Sideral Time":string)  [unwired: 1 in, 2 out]
              }
              frame #1 {
                # "OV 2024 09 04: Depois da criação da aba CCD modes, TODOS os parametros da aba Camera são protegidos por senha, \ninclusive as chaves de habilitação dos canais."
                n164 = Unbundle By Name(w386) -> ("S4ICS id"=w384:u32)
                n165 = Unbundle By Name(w382) -> ("Cluster AdmCCDsetup.param"=w379:T12)
                n166 = Equal?(x=u32 11, y=w384) -> (x = y?=w383:bool)
                n167 = local write "S4ICS protocol"(w383) -> ()
                n168 = case shown="\"Disabled and Grayed Out\"" w379 {
                  tunnel: [_ w388 w392] -> w381
                  frame Default {
                  }
                  frame "Disabled" {
                    n169 = Build Array(u32 4 ("element"), u32 5 ("element"), u32 6 ("element")) -> (w388:u32[])
                  }
                  frame "Disabled and Grayed Out" {
                    n170 = Build Array(u32 4 ("element"), u32 5 ("element"), u32 6 ("element")) -> (w392:u32[])
                  }
                }
                n171 = property on="Trigger\nMode" class="Ring (strict)"("DisabledEnum"=w379) -> ()  [unwired: 2 in, 2 out]
                n172 = property on="Vertical\nShift Speed" class="Ring (strict)"("DisabledEnum"=w379) -> ()  [unwired: 2 in, 2 out]
                n173 = property on="Vertical\nClock Voltage" class="Ring (strict)"("DisabledEnum"=w379) -> ()  [unwired: 2 in, 2 out]
                n174 = To Long Integer(number=w381) -> (32bit integer=w380:i32[])
                n175 = property on="EM Gain" class="DigNum (strict)"("DisabledEnum"=w379) -> ()  [unwired: 2 in, 2 out]
                n176 = property on="Read\nMode" class="Ring (strict)"("DisabledEnum"=w379) -> ()  [unwired: 2 in, 2 out]
                n177 = property on="AQM" class="Enum (strict)"("Disabled Items []"=w380) -> ()  [unwired: 2 in, 2 out]
                n178 = property on="Acquisition\nMode" class="Ring (strict)"("DisabledEnum"=w379) -> ()  [unwired: 2 in, 2 out]
                n179 = property on="A/D \nChannel" class="DigNum (strict)"("DisabledEnum"=w379) -> ()  [unwired: 2 in, 2 out]
                n180 = property on="Readout\nRate" class="Ring (strict)"("DisabledEnum"=w379) -> ()  [unwired: 2 in, 2 out]
                n181 = property on="CCD \nEM Mode" class="Ring (strict)"("DisabledEnum"=w379) -> ()  [unwired: 2 in, 2 out]
                n182 = property on="CCD\nEM Gain" class="DigNum (strict)"("DisabledEnum"=w379) -> ()  [unwired: 2 in, 2 out]
                n183 = property on="Shutter\nTTL" class="Ring (strict)"("DisabledEnum"=w379) -> ()  [unwired: 2 in, 2 out]
                n184 = property on="Shutter\nOpenning Time" class="DigNum (strict)"("DisabledEnum"=w379) -> ()  [unwired: 2 in, 2 out]
                n185 = property on="Frame\nTransfer" class="Bool (strict)"("DisabledEnum"=w379) -> ()  [unwired: 2 in, 2 out]
                n186 = property on="Shutter\nMode" class="Ring (strict)"("DisabledEnum"=w379) -> ()  [unwired: 2 in, 2 out]
                n187 = property on="Pre-amplification\nGain" class="Ring (strict)"("DisabledEnum"=w379) -> ()  [unwired: 2 in, 2 out]
                n188 = property on="Shutter\nClosing Time" class="DigNum (strict)"("DisabledEnum"=w379) -> ()  [unwired: 2 in, 2 out]
                n189 = property on="Horizontal\nBinning" class="DigNum (strict)"("DisabledEnum"=w379) -> ()  [unwired: 2 in, 2 out]
                n190 = property on="Vertical\nBinning" class="DigNum (strict)"("DisabledEnum"=w379) -> ()  [unwired: 2 in, 2 out]
                n191 = property on="Image\nFInal Column" class="DigNum (strict)"("DisabledEnum"=w379) -> ()  [unwired: 2 in, 2 out]
                n192 = property on="CH1on" class="Bool (strict)"("DisabledEnum"=w379) -> ()  [unwired: 2 in, 2 out]
                n193 = property on="CH2on" class="Bool (strict)"("DisabledEnum"=w379) -> ()  [unwired: 2 in, 2 out]
                n194 = property on="CH3 on" class="Bool (strict)"("DisabledEnum"=w379) -> ()  [unwired: 2 in, 2 out]
                n195 = property on="CH4 on" class="Bool (strict)"("DisabledEnum"=w379) -> ()  [unwired: 2 in, 2 out]
                n196 = property on="Image\nFinal Line" class="DigNum (strict)"("DisabledEnum"=w379) -> ()  [unwired: 2 in, 2 out]
                n197 = property on="Image\nInitial Column" class="DigNum (strict)"("DisabledEnum"=w379) -> ()  [unwired: 2 in, 2 out]
                n198 = property on="Image \nInitial Line" class="DigNum (strict)"("DisabledEnum"=w379) -> ()  [unwired: 2 in, 2 out]
              }
              frame #2 {
                n199 = Unbundle By Name(w398) -> ("Trigger Mode Status"=→"String":string, "Focus_connection"=→"Focus 160":bool, "WS_connection"=→"Weather":bool)
              }
              frame #3 {
                n200 = Unbundle By Name(w400) -> ("Trigger General Status"=→"String 2":string)
              }
              frame #4 {
                n201 = Unbundle By Name(w407) -> ("Instrument Status"=w401:T18, "Instrument States.WPROT State"=w406:i32, "Instrument Pos Names.WPROT posname"=w405:string, "Instrument Pos Names.WPSEL posname"=w404:string, "Instrument Pos Names.CALW posname"=w403:string, "Instrument Pos Names.ASEL posname"=w402:string)
                n202 = stacked-sequence {
                  tunnel: w401 -> [w414 w417 w420 w422 w424 w427 w430 w436 w438]
                  tunnel: w406 -> [w410 _ _ _ _ _ _ _ _]
                  tunnel: w405 -> [_ w415 _ _ _ _ _ _ _]
                  tunnel: w404 -> [_ _ w418 _ _ _ _ _ _]
                  tunnel: w403 -> [_ _ _ _ _ w425 _ _ _]
                  tunnel: w402 -> [_ _ _ _ _ _ w428 _ _]
                  frame #0 {
                    # "Pisca quando BUSY"
                    n203 = Unbundle By Name(w414) -> ("WPROT pos"=w411:dbl)
                    "WaveplatePos 2" <- w411
                    n204 = Equal?(x=w410, y=3) -> (x = y?=w408:bool)
                    n205 = property on="WaveplatePos 2" class="DigNum (strict)"("Blinking"=w408) -> ()  [unwired: 2 in, 2 out]
                    n206 = Number To Fractional String(number=w411, precision (6)=i16 1) -> (F-format string=→"Angle":string)  [unwired: 2 in]
                  }
                  frame #1 {
                    n207 = Unbundle By Name(w417) -> ("WPROT pos"=→"Position WPROT":dbl)
                    "PosName WPROT" <- w415
                  }
                  frame #2 {
                    n208 = Unbundle By Name(w420) -> ("WPSEL pos"=→"Position WPSEL":dbl)
                    "PosName WPSEL" <- w418
                  }
                  frame #3 {
                    n209 = Unbundle By Name(w422) -> ("GMIR pos"=→"Position GMIR":dbl)
                  }
                  frame #4 {
                    n210 = Unbundle By Name(w424) -> ("GFOC pos"=→"Position GFOC":dbl)
                  }
                  frame #5 {
                    n211 = Unbundle By Name(w427) -> ("CALW pos"=→"Position CALW":dbl)
                    "PosName CALW" <- w425
                  }
                  frame #6 {
                    n212 = Unbundle By Name(w430) -> ("ASEL pos"=→"PosName ASEL":dbl)
                    "PosName ASEL" <- w428
                  }
                  frame #7 {
                    w432 = cluster{u32, u32}[] [{16711680, 16711680}, {15400704, 15400704}, {16776722, 0}, {16776722, 0}]  # amarelo
                    w431 = cluster{u32, u32}[] [{16711680, 16711680}, {6618880, 6618880}, {16776722, 0}, {16776722, 0}]  # verde
                    n213 = Unbundle By Name(w436) -> ("connection"=→"S4ICSoft":bool, "operational"=w434:bool)
                    n214 = Select(t=w431, s=w434, f=w432) -> (s? t:f=w433:cluster{u32, u32}[])
                    n215 = property on="S4ICSoft" class="Bool (strict)"("Colors [4]"=w433) -> ()  [unwired: 2 in, 2 out]
                  }
                  frame #8 {
                    n216 = Unbundle By Name(w438) -> ("String Status"=→"Status":string)
                  }
                }
              }
              frame #5 {
                n217 = Unbundle By Name(w441) -> ("Sync Box State"=→"Current State":i32, "Trigger_connection"=→"Sync Box" →"LedExtSync":bool)
              }
              frame #6 {
                # "Instrument States.<device> State\n\n0: nao fez INIT e está parado (mode = IDLE ou WAITING\n                                                    contdition = default)\n1: nao fez INIT e está movendo (mode = IDLE ou WAITING\n                                                    contdition = BUSY)\n\n2: fez INIT e está parado (mode = default)\n                                            condition = READY)\n3: fez INIT e está movendo (mode = default)\n                                            condition = BUSY)"
                n218 = Unbundle By Name(w444) -> ("Instrument States"=w443:T19, "Instrument Pos Names"=w442:T20)
                n219 = stacked-sequence {
                  tunnel: w443 -> [w452 w474 w492 w526 w551 w565]
                  tunnel: w442 -> [w448 _ w490 w522 _ _]
                  frame #0 {
                    # "WPSEL"
                    n220 = Unbundle By Name(w448) -> ("WPSEL posname"=w445:string)
                    n221 = Unbundle By Name(w452) -> ("WPSEL State"=w451:i32)
                    n222 = local read "WPSEL Status"() -> (w447:bool)
                    n223 = case shown="2" w451 {
                      tunnel: [cluster{u32, u32}[] [{9868950, 9868950}, {9868950, 9868950}] ("Colors [4]") cluster{u32, u32}[] [{9868950, 9868950}, {9868950, 9868950}] ("Colors [4]") cluster{u32, u32}[] [{16318208, 16318208}, {16318208, 16318208}] ("Colors [4]") cluster{u32, u32}[] [{6618880, 2424594}, {6618880, 2424594}] ("Colors [4]") w466] -> w450
                      tunnel: [FALSE ("WPROT Status") FALSE ("WPROT Status") TRUE ("WPROT Status") FALSE ("WPROT Status") w468] -> w449
                      tunnel: w447 -> [_ _ _ _ w467]
                      tunnel: ["" "" "" w462 ""] -> w446
                      tunnel: w445 -> [_ _ _ w462 _]
                      frame Default {
                      }
                      frame 0 {
                      }
                      frame 1 {
                      }
                      frame 2 {
                      }
                      frame 3 {
                        n224 = case shown="True" w467 {
                          tunnel: [cluster{u32, u32}[] [{7563008, 7563008}, {7563008, 7563008}] ("Colors [4]") cluster{u32, u32}[] [{16318208, 16318208}, {16318208, 16318208}] ("Colors [4]")] -> w466
                          frame False {
                          }
                          frame True {
                          }
                        }
                        n225 = Not(x=w467) -> (.not. x?=w468:bool)
                      }
                    }
                    "WPSEL Status" <- w449
                    "Waveplate" <- w449
                    n226 = property on="Waveplate" class="Bool (strict)"("Colors [4]"=w450, "BoolText.Text"=w446) -> ()  [unwired: 2 in, 2 out]
                    n227 = property on="WPSEL Status" class="Bool (strict)"("Colors [4]"=w450) -> ()  [unwired: 2 in, 2 out]
                  }
                  frame #1 {
                    # "WPROT"
                    n228 = Unbundle By Name(w474) -> ("WPROT State"=w473:i32)
                    n229 = case shown="2" w473 {
